vi "GetPositionSetting.vi"(10 "基路径":path=path "C:/Labview Code/System/Part Configuration", 11 "Part Type":string) -> (3 "Hall Positions":i32[](array[numeric]))   [LabVIEW 2018]
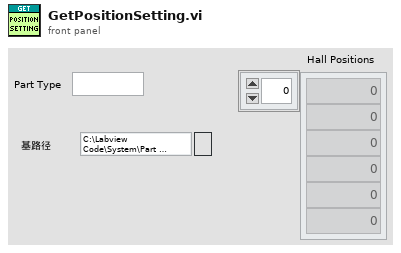
[diagram p1: front panel]
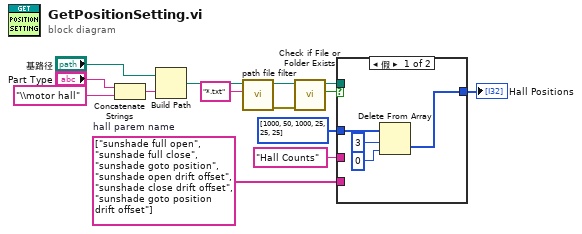
[diagram p0: block diagram]
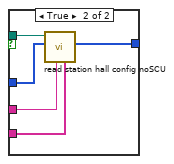
[diagram p2: hidden frame]
diagram:
  w3 = string[] ["sunshade full open", "sunshade full close", "sunshade goto position", "sunshade open drift offset", "sunshade close drift offset", "sunshade goto position drift offset"]  # hall parem name
  n1 = Concatenate Strings("Part Type", "\\motor hall" ("string")) -> (w12:string)
  n2 = Build Path(base path="基路径", name or relative path=w12) -> (appended path=w14:path)
  n3 = call "path file filter.vi"("file type"="*.txt", "path"=w14) -> ("错误输出"=w11:errorcluster, "File path"=w10:path)  [unwired: 8 in]
  n4 = call <vilib>:"Check if File or Folder Exists.vi"("error in (no error)"=w11, "path"=w10) -> ("file or folder exists?"=w6:bool, "dup path"=w5:path)  [unwired: 7 in, 1 out]
  n5 = case shown="假" w6 {
    tunnel: w5 -> [_ w23]
    tunnel: i32[] [1000, 50, 1000, 25, 25, 25] ("Hall Positions") -> [w18 w22]
    tunnel: w3 -> [_ w21]
    tunnel: "Hall Counts" ("section") -> [_ w20]
    tunnel: [w16 w19] -> w1
    frame False {
      n6 = Delete From Array(array=w18, length=3 ("长度"), index=0 ("索引")) -> (deleted portion=w16:i32[])  [unwired: 1 out]
    }
    frame True {
      n7 = call "read station hall config noSCU.vi"("name"=w21, "section"=w20, "default value"=w22, "configuration file path in"=w23) -> ("Hall Positions"=w19:i32[])  [unwired: 4 in, 3 out]
    }
  }
  "Hall Positions" <- w1
